vi "Apply UW Offset to Tun Coordinates.vi"(1 "Traverse Name":string, 2 "Tunnel Coordinates":sgl[](array[numeric])) -> (0 "UW Offset Applied":sgl[](array[numeric]))   [LabVIEW 2018]
uses:
  Globals/Trav_pos_global.vi
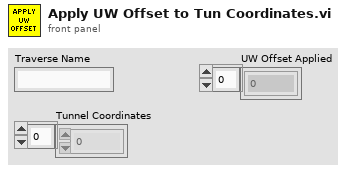
[diagram p1: front panel]
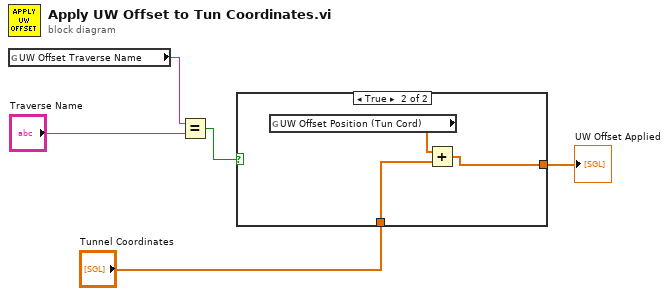
[diagram p0: block diagram]
diagram:
  n1 = global read "Trav_pos_global.vi" "UW Offset Traverse Name"() -> (w1:string)
  n2 = Equal?(x=w1, y="Traverse Name") -> (x = y?=w3:bool)
  n3 = case shown="True" w3 {
    tunnel: "Tunnel Coordinates" -> [w6 w8]
    tunnel: [w6 w7] -> w5
    frame False {
    }
    frame True {
      n4 = global read "Trav_pos_global.vi" "UW Offset Position (Tun Cord)"() -> (w9:sgl[])
      n5 = Add(x=w9, y=w8) -> (x+y=w7:sgl[])
    }
  }
  "UW Offset Applied" <- w5
